vi "recipe_logic.vi"(5 "waitgroup":T3, 7 "references":T1, 8 "error in (no error)":errorcluster, 11 "data_in":T4) -> (0 "error out":errorcluster, 1 "data":variant, 2 "change":bool, 3 "data_out":T4)   [LabVIEW 2015, in "lv-recipe-machine.lvlib"]
uses:
  lv-recipe-machine.lvlib
  _controls/recipe_data.ctl
  public/_controls/mode.ctl
  public/_controls/manual_state.ctl
  public/_controls/automatic_state.ctl
  <userlib>/antonio-alexander/lv-waitgroup/public/_controls/api_waitgroup.ctl
  lv-recipe-machine_/public/_controls/references.ctl
  lv-recipe-machine_/private/_controls/input.ctl
  lv-recipe-machine_/private/_controls/input_command.ctl
  lv-recipe-machine_/private/_controls/output.ctl
  lv-recipe-machine_/private/_controls/data.ctl
  lv-recipe-machine_/public/_controls/configuration.ctl
  public/_controls/transition.ctl
  lv-recipe-machine_/public/_controls/change.ctl
  public/_controls/step.ctl
  public/_controls/step_vi_reference.ctl
  <vilib>/ptbypt/NI_PtbyPt.lvlib
  <userlib>/antonio-alexander/lv-waitgroup/lv-waitgroup.lvlib
  lv-recipe-machine_/repub-dvr_nre.lvlib
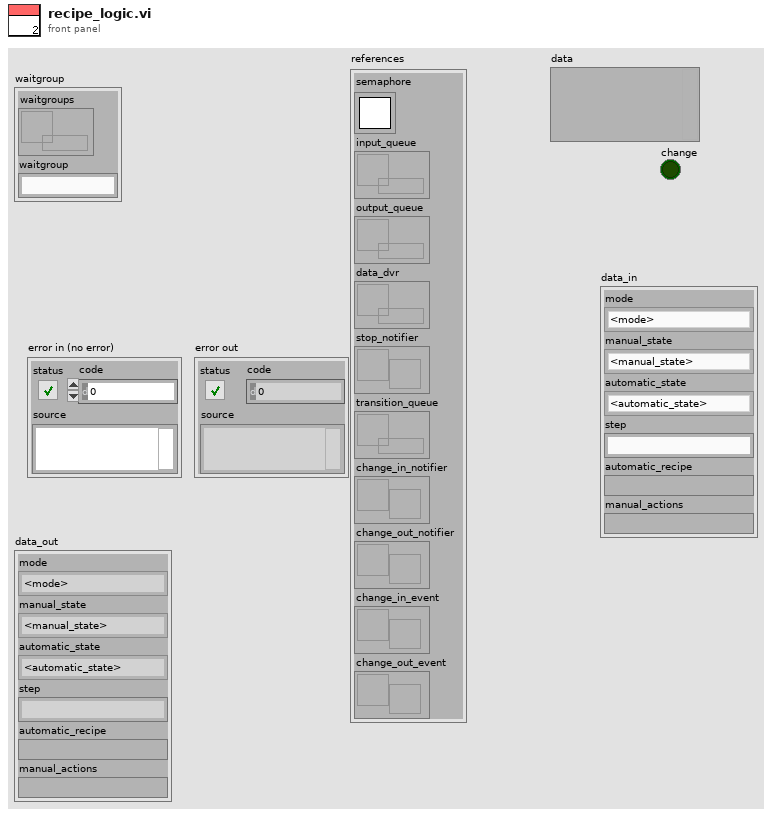
[diagram p1: front panel]
types:
  T1 = typedef "repub-dvr_nre.lvlib/references.ctl" = cluster{"semaphore":T2, "input_queue":refnum<queue>, "output_queue":refnum<queue>, "data_dvr":refnum<data-value>, "stop_notifier":refnum<notifier>, "transition_queue":refnum<queue>, "change_in_notifier":refnum<notifier>, "change_out_notifier":refnum<notifier>, "change_in_event":refnum<user-event>, "change_out_event":refnum<user-event>}
  T2 = typedef "Semaphore RefNum" = refnum<k1>
  T3 = typedef "lv-waitgroup.lvlib/api_waitgroup.ctl" = cluster{"waitgroups":refnum<data-value>, "waitgroup":string}
  T4 = typedef "lv-recipe-machine.lvlib/recipe_data.ctl" = cluster{"mode":T5, "manual_state":T6, "automatic_state":T7, "step":string, "automatic_recipe":variant, "manual_actions":variant}
  T5 = typedef "lv-recipe-machine.lvlib/mode.ctl" = enum16{"<mode>", "manual", "automatic", "<null>"}
  T6 = typedef "lv-recipe-machine.lvlib/manual_state.ctl" = enum16{"<manual_state>", "failed", "action", "running", "idle", "<null>"}
  T7 = typedef "lv-recipe-machine.lvlib/automatic_state.ctl" = enum16{"<automatic_state>", "failed", "idle", "running", "paused", "transition", "stopped", "<null>"}
  T8 = typedef "lv-recipe-machine.lvlib/step.ctl" = cluster{"name":string, "step_vi_reference":T9, "data":variant}
  T9 = typedef "lv-recipe-machine.lvlib/step_vi_reference.ctl" = refnum<vi>
  T10 = typedef "lv-recipe-machine.lvlib/transition.ctl" = cluster{"next_step":string, "data":variant, "error":errorcluster}
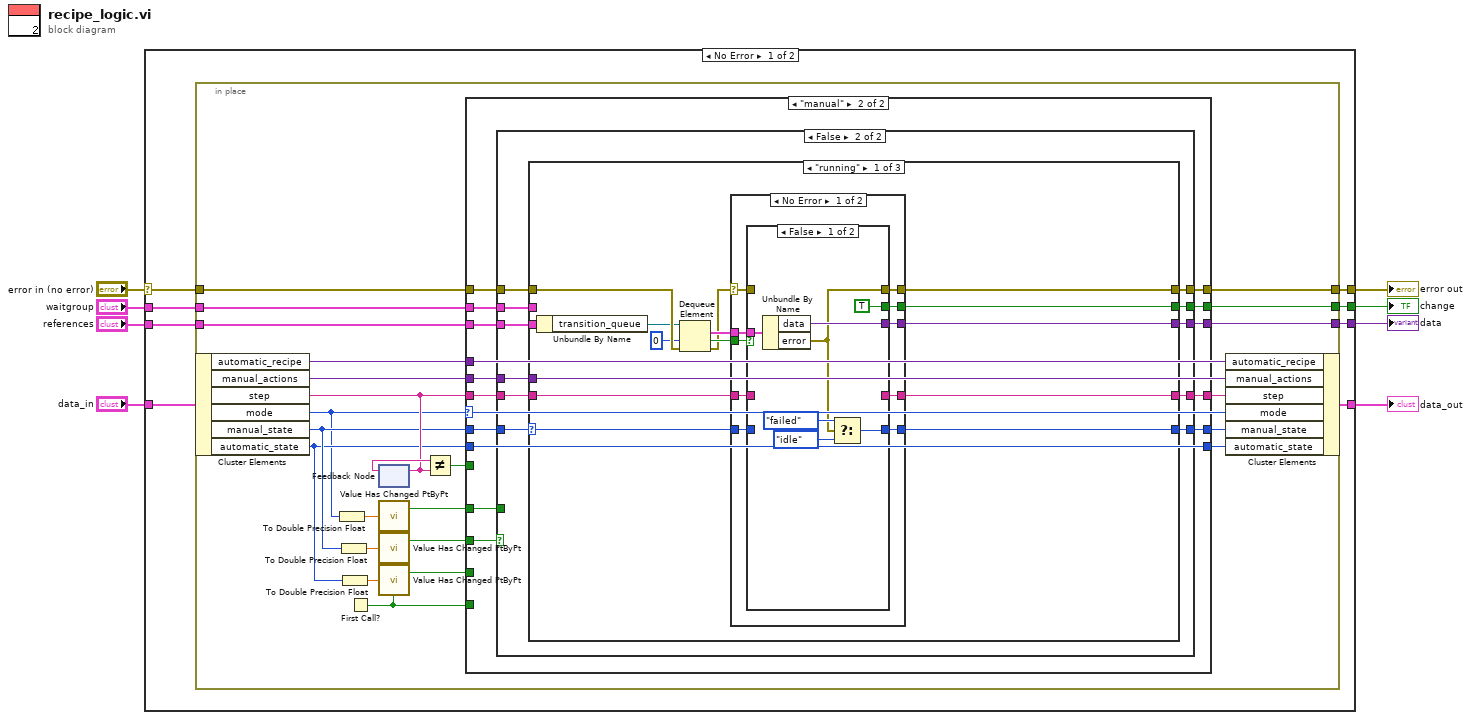
[diagram p0: block diagram]
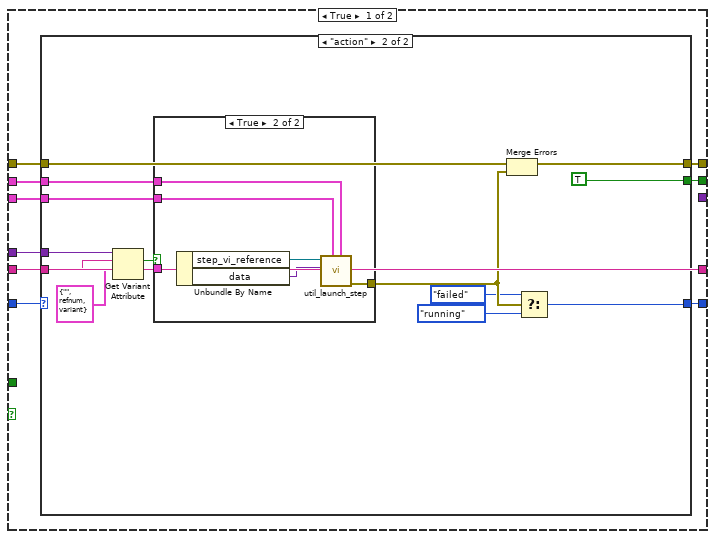
[diagram p3: hidden frame]
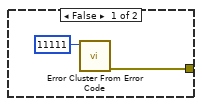
[diagram p5: hidden frame]
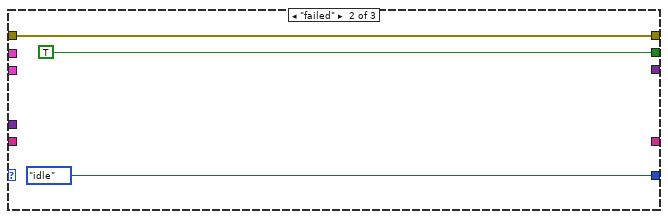
[diagram p8: hidden frame]
diagram:
  n1 = case shown="No Error" "error in (no error)" {
    selector: "error in (no error)" -> [w16 w147]
    tunnel: [w12 w147] -> w7
    tunnel: "data_in" -> [w15 w146]
    tunnel: "waitgroup" -> [w14 _]
    tunnel: [w13 w146] -> w4
    tunnel: "references" -> [w11 _]
    tunnel: [w10 _] -> w3
    tunnel: [w9 _] -> w2
    frame No Error {
      n2 = in-place {
        in-place-border: w16 -> [w32]
        in-place-border: w14 -> [w30]
        in-place-border: [w26] -> w12
        in-place-border: w11 -> [w20]
        in-place-border: [w18] -> w10
        in-place-border: [w17] -> w9
        n3 = in-place-cluster #1(w15) -> ("automatic_recipe"=w21:variant, "manual_actions"=w19:variant, "step"=w29:string, "mode"=w24:T5, "manual_state"=w28:T6, "automatic_state"=w27:T7)
        n4 = To Double Precision Float(number=w24) -> (double precision float=w40:dbl)
        n5 = To Double Precision Float(number=w28) -> (double precision float=w39:dbl)
        n6 = To Double Precision Float(number=w27) -> (double precision float=w38:dbl)
        n7 = First Call?() -> (First Call?: T/F=w31:bool)
        n8 = feedback #2() -> (w34:string)  [unwired: 1 in]
        n9 = feedback-in #2(w29) -> ()
        n10 = call <vilib>:"Value Has Changed PtByPt.vi"("input data point"=w40, "initialize"=w31) -> ("has changed"=w37:bool)  [unwired: 1 out]
        n11 = call <vilib>:"Value Has Changed PtByPt.vi"("input data point"=w39, "initialize"=w31) -> ("has changed"=w36:bool)  [unwired: 1 out]
        n12 = call <vilib>:"Value Has Changed PtByPt.vi"("input data point"=w38, "initialize"=w31) -> ("has changed"=w35:bool)  [unwired: 1 out]
        n13 = Not Equal?(x=w34, y=w29) -> (x != y?=w33:bool)
        n14 = case shown="\"manual\"" w24 {
          tunnel: w28 -> [w42 w58]
          tunnel: w27 -> [w41 w48]
          tunnel: w37 -> [_ w57]
          tunnel: w36 -> [_ w56]
          tunnel: w35 -> [_ _]
          tunnel: w31 -> [_ _]
          tunnel: w21 -> [_ _]
          tunnel: w29 -> [w43 w55]
          tunnel: w33 -> [_ _]
          tunnel: w32 -> [w44 w53]
          tunnel: w30 -> [_ w54]
          tunnel: [w44 w52] -> w26
          tunnel: [w43 w49] -> w25
          tunnel: [w42 w51] -> w23
          tunnel: [w41 w48] -> w22
          tunnel: w19 -> [_ w50]
          tunnel: w20 -> [_ w47]
          tunnel: [_ w46] -> w18
          tunnel: [_ w45] -> w17
          frame Default {
          }
          frame "manual" {
            n15 = case shown="False" w56 {
              tunnel: w57 -> [_ _]
              tunnel: w58 -> [w67 w102]
              tunnel: w55 -> [w61 w101]
              tunnel: w54 -> [w66 w100]
              tunnel: w53 -> [w65 w99]
              tunnel: [w64 w98] -> w52
              tunnel: [w63 w97] -> w51
              tunnel: w50 -> [w62 w96]
              tunnel: [w61 w95] -> w49
              tunnel: w47 -> [w60 w94]
              tunnel: [w59 w93] -> w46
              tunnel: [_ w92] -> w45
              frame True {
                n16 = case shown="\"action\"" w67 {
                  selector: w67 -> [w68 _]
                  tunnel: w61 -> [_ w83]
                  tunnel: w66 -> [_ w80]
                  tunnel: w65 -> [w69 w79]
                  tunnel: [w69 w77] -> w64
                  tunnel: [w68 w73] -> w63
                  tunnel: w62 -> [_ w72]
                  tunnel: w60 -> [_ w71]
                  tunnel: [_ TRUE] -> w59
                  frame Default {
                  }
                  frame "action" {
                    n17 = Get Variant Attribute(Variant=w72, name=w83, default value (empty Variant)=T8 {"name"="", "step_vi_reference"=refnum, "data"=variant} ("step")) -> (found=w78:bool, value=w81:T8)  [unwired: 1 in, 2 out]
                    n18 = case shown="True" w78 {
                      tunnel: w81 -> [_ w91]
                      tunnel: w80 -> [_ w87]
                      tunnel: [w85 w90] -> w76
                      tunnel: w71 -> [_ w86]
                      frame False {
                        n19 = call <vilib>:"Error Cluster From Error Code.vi"("error code (0)"=11111) -> ("error out"=w85:errorcluster)  [unwired: 8 in]
                      }
                      frame True {
                        n20 = Unbundle By Name(w91) -> ("step_vi_reference"=w89:T9, "data"=w88:variant)
                        n21 = call "util_launch_step.vi"("waitgroup"=w87, "references"=w86, "data"=w88, "step_vi_reference"=w89) -> ("error out"=w90:errorcluster)  [unwired: 7 in]
                      }
                    }
                    n22 = Merge Errors(w79, w76) -> (w77:errorcluster)
                    n23 = Select(t=manual_state."failed" ("manual_state"), s=w76, f=manual_state."running" ("manual_state")) -> (s? t:f=w73:T6)
                  }
                }
              }
              frame False {
                n24 = case shown="\"running\"" w102 {
                  selector: w102 -> [w110 _ w143]
                  tunnel: w101 -> [w112 _ w144]
                  tunnel: w100 -> [_ _ _]
                  tunnel: w99 -> [w116 w141 w145]
                  tunnel: [w105 w141 w145] -> w98
                  tunnel: [w111 manual_state."idle" ("manual_state") w143] -> w97
                  tunnel: w96 -> [_ _ _]
                  tunnel: [w108 _ w144] -> w95
                  tunnel: w94 -> [w104 _ _]
                  tunnel: [w107 TRUE _] -> w93
                  tunnel: [w106 _ _] -> w92
                  frame "running" {
                    n25 = Unbundle By Name(w104) -> ("transition_queue"=w103:refnum<queue>)
                    n26 = Dequeue Element(queue=w103, timeout in ms (-1)=0, error in (no error)=w116) -> (element=w114:T10, timed out?=w113:bool, error out=w109:errorcluster)  [unwired: 1 out]
                    n27 = case shown="No Error" w109 {
                      selector: w109 -> [w117 w137]
                      tunnel: w114 -> [w126 _]
                      tunnel: w113 -> [w125 _]
                      tunnel: w112 -> [w124 w138]
                      tunnel: [w123 w139] -> w111
                      tunnel: w110 -> [w122 w139]
                      tunnel: [w121 w138] -> w108
                      tunnel: [w120 _] -> w107
                      tunnel: [w119 _] -> w106
                      tunnel: [w118 w137] -> w105
                      frame No Error {
                        n28 = case shown="False" w125 {
                          tunnel: w126 -> [w133 _]
                          tunnel: w124 -> [_ w135]
                          tunnel: [w132 w136] -> w123
                          tunnel: w122 -> [_ w136]
                          tunnel: [_ w135] -> w121
                          tunnel: [TRUE _] -> w120
                          tunnel: [w128 _] -> w119
                          tunnel: [w127 w134] -> w118
                          tunnel: w117 -> [_ w134]
                          frame False {
                            n29 = Unbundle By Name(w133) -> ("data"=w128:variant, "error"=w127:errorcluster)
                            n30 = Select(t=manual_state."failed" ("manual_state"), s=w127, f=manual_state."idle" ("manual_state")) -> (s? t:f=w132:T6)
                          }
                          frame True {
                          }
                        }
                      }
                      frame Error {
                      }
                    }
                  }
                  frame "failed" {
                  }
                  frame Default {
                  }
                }
              }
            }
          }
        }
        n31 = in-place-cluster #1("automatic_recipe"=w21, "manual_actions"=w19, "step"=w25, "mode"=w24, "manual_state"=w23, "automatic_state"=w22) -> (w13:T4)
      }
    }
    frame Error {
    }
  }
  "error out" <- w7
  "data_out" <- w4
  "change" <- w3
  "data" <- w2
